vi "Run Test.vi"(8 "error in (no error)":errorcluster, 11 "CCT Test in":refnum<class "CTT Power-Up Test.lvclass">) -> (0 "error out":errorcluster, 1 "Fail Codes":string[](array[string]), 2 "Tests Passed":bool[](array[boolean]), 3 "CCT Test out":refnum<class "CTT Power-Up Test.lvclass">)   [LabVIEW 2015, in "CTT Power-Up Test.lvclass"]
uses:
  CTT Power-Up Test.lvclass
  Test Class/Test Class.lvclass
  Classes/Application/Class/Application.lvclass
  CT Common Tests/CT Common Tests.lvclass
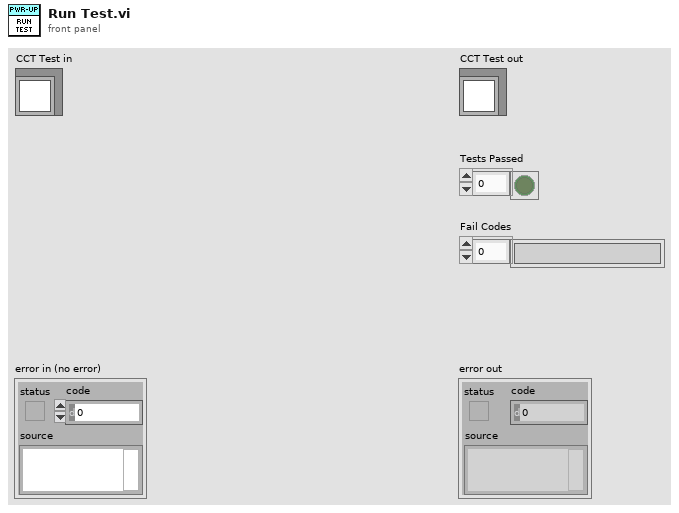
[diagram p1: front panel]
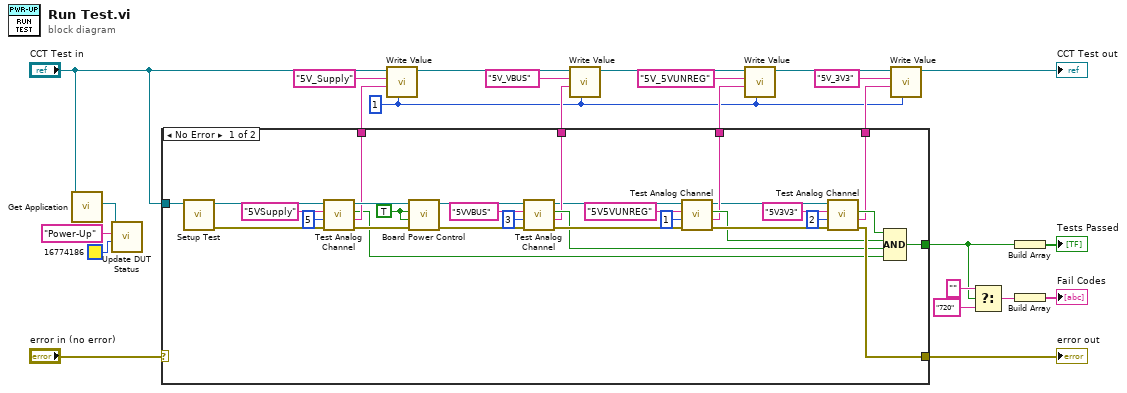
[diagram p0: block diagram]
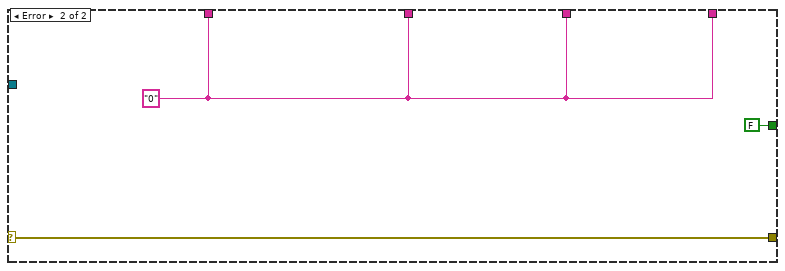
[diagram p2: hidden frame]
diagram:
  w16 = 1 ("DUT")
  n1 = call "Get Application.vi"("Test Class in"="CCT Test in") -> ("Application.lvlib:Application.lvclass"=w6:refnum<class "Application.lvclass">)  [unwired: 9 in, 1 out]
  n2 = call "Update DUT Status.vi"("BG Color"=u32 16774186, "Message ('')"="Power-Up", "Application in"=w6) -> ()  [unwired: 7 in, 2 out]
  n3 = case shown="No Error" "error in (no error)" {
    selector: "error in (no error)" -> [_ w54]
    tunnel: [w51 w54] -> w21
    tunnel: [w46 FALSE] -> w10
    tunnel: [w41 w53] -> w20
    tunnel: [w35 w53] -> w19
    tunnel: [w30 w53] -> w18
    tunnel: [w25 w53] -> w17
    tunnel: "CCT Test in" -> [w45 _]
    frame No Error {
      w39 = TRUE ("Power-On")
      n4 = call "Setup Test.vi"("CTT Power-Up Test"=w45) -> ("error out"=w50:errorcluster, "CTT Power-Up Test"=w24:refnum<class "CTT Power-Up Test.lvclass">)  [unwired: 9 in]
      n5 = call "Test Analog Channel.vi"("error in (no error)"=w50, "Channel (0)"=u32 5, "Test Label"="5VSupply", "CT Common Tests in"=w24) -> ("error out"=w49:errorcluster, "Result"=w41:string, "Passed"=w40:bool, "CT Common Tests out"=w42:refnum<class "CTT Power-Up Test.lvclass">)  [unwired: 4 in]
      n6 = call "Board Power Control.vi"("error in (no error)"=w49, "VBUS"=w39, "Power-On"=w39, "CT Common Tests"=w42) -> ("error out"=w22:errorcluster, "CT Common Tests"=w23:refnum<class "CTT Power-Up Test.lvclass">)  [unwired: 6 in]
      n7 = call "Test Analog Channel.vi"("error in (no error)"=w22, "Channel (0)"=u32 3, "Test Label"="5VVBUS", "CT Common Tests in"=w23) -> ("error out"=w48:errorcluster, "Result"=w35:string, "Passed"=w36:bool, "CT Common Tests out"=w34:refnum<class "CTT Power-Up Test.lvclass">)  [unwired: 4 in]
      n8 = call "Test Analog Channel.vi"("error in (no error)"=w48, "Channel (0)"=u32 1, "Test Label"="5V5VUNREG", "CT Common Tests in"=w34) -> ("error out"=w47:errorcluster, "Result"=w30:string, "Passed"=w31:bool, "CT Common Tests out"=w29:refnum<class "CTT Power-Up Test.lvclass">)  [unwired: 4 in]
      n9 = call "Test Analog Channel.vi"("error in (no error)"=w47, "Channel (0)"=u32 2, "Test Label"="5V3V3", "CT Common Tests in"=w29) -> ("error out"=w51:errorcluster, "Result"=w25:string, "Passed"=w26:bool)  [unwired: 4 in, 1 out]
      n10 = Compound Arithmetic op=AND(w26, w31, w36, w40) -> (w46:bool)
    }
    frame Error {
      w53 = "0" ("Test Label")
    }
  }
  "error out" <- w21
  n11 = call "Write Value.vi"("Position"=w16, "Value"=w20, "Label"="5V_Supply" ("Test Label"), "Test Class in"="CCT Test in") -> ()  [unwired: 7 in, 1 out]
  n12 = call "Write Value.vi"("Position"=w16, "Value"=w19, "Label"="5V_VBUS" ("Test Label"), "Test Class in"="CCT Test in") -> ()  [unwired: 7 in, 1 out]
  n13 = call "Write Value.vi"("Position"=w16, "Value"=w18, "Label"="5V_5VUNREG" ("Test Label"), "Test Class in"="CCT Test in") -> ()  [unwired: 7 in, 1 out]
  n14 = call "Write Value.vi"("Position"=w16, "Value"=w17, "Label"="5V_3V3" ("Test Label"), "Test Class in"="CCT Test in") -> ()  [unwired: 7 in, 1 out]
  n15 = Select(t="", s=w10, f="720") -> (s? t:f=w14:string)
  n16 = Build Array(w10) -> (→"Tests Passed":bool[])
  n17 = Build Array(w14) -> (→"Fail Codes":string[])
  "CCT Test out" <- "CCT Test in"
